vi "FPGA Interleaving.vi"() -> ()   [LabVIEW 2010]
uses:
  <vilib>/LabVIEW Targets/FPGA/cRIO/shared/nicrio_ModuleControls/nicrio_cRIO-9233_DataRatesRing.ctl
  <vilib>/eio/EIOPropertyNode/EIOPropertyNode.xnode
  <vilib>/rvi/eio/nirviEIOPropertyImplementation/nirviEIOPropertyImplementation.xnode
  <vilib>/eio/EIONode/EIONode.xnode
  <vilib>/rvi/eio/nirviEIOImplementation/nirviEIOImplementation.xnode
  <vilib>/rvi/eio/common/nirviEmuClasses.ctl
  <vilib>/rvi/DataTransferAndStorage/Container/XNode/niFpgaContainer.xnode
  <vilib>/rvi/DataTransferAndStorage/Container/Common/niFpgaContainerMethod.ctl
  <vilib>/rvi/DataTransferAndStorage/Container/Common/niFpgaTransferTypeControl.ctl
  <vilib>/rvi/eio/common/nirviEmuTemplatePropertySet_noerrors.vi
  <vilib>/rvi/eio/common/nirviEmuTemplateMethod_noerrors.vi
  <vilib>/rvi/interface/RandomDataEmulation/nirviRandomDataFPGAFIFO.vi
  <vilib>/rvi/interface/RandomDataEmulation/niFpgaRandomDataHandleErrors.vi
panel:
  in  "Samples per Channel":i32
  in  "Data Rate":T1=57 items=["50.000 kS/s (NI 9233)"=2, "33.333 kS/s (NI 9233)"=3, "25.000 kS/s (NI 9233)"=34, "16.667 kS/s (NI 9233)"=35, "12.500 kS/s (NI 9233)"=36, "10.000 kS/s (NI 9233)"=37, "  8.333 kS/s (NI 9233)"=38, "  7.143 kS/s (NI 9233)"=39, "  6.250 kS/s (NI 9233)"=40, "  5.556 kS/s (NI 9233)"=41, "  5.000 kS/s (NI 9233)"=42, "  4.545 kS/s (NI 9233)"=43, "  4.167 kS/s (NI 9233)"=44, "  3.846 kS/s (NI 9233)"=45, "  3.571 kS/s (NI 9233)"=46, "  3.333 kS/s (NI 9233)"=47, "  3.125 kS/s (NI 9233)"=48, "  2.941 kS/s (NI 9233)"=49, "  2.778 kS/s (NI 9233)"=50, "  2.632 kS/s (NI 9233)"=51, "  2.500 kS/s (NI 9233)"=52, "  2.381 kS/s (NI 9233)"=53, "  2.273 kS/s (NI 9233)"=54, "  2.174 kS/s (NI 9233)"=55, "  2.083 kS/s (NI 9233)"=56, "  2.000 kS/s (NI 9233)"=57]
  out "Overflow Occurred":bool
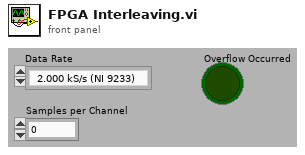
[diagram p1: front panel]
types:
  T1 = typedef "nicrio_cRIO-9233_DataRatesRing.ctl" = u8
  T2 = typedef "nirviEmuClasses.ctl" = enum16{"IO Read", "IO Write", "Method", "Property Read", "Property Write"}
  T3 = typedef "niFpgaContainerMethod.ctl" = enum16{"<none>", "write", "read", "clear", "getNumberOfElementsToWrite", "getNumberOfElementsToRead", "enable", "disable", "flushAndDisable", "getStreamState", "readA", "readB", "dramWrite", "dramWriteWithByteEnables", "dramRequestData", "dramRetrieveData"}
  T4 = typedef "niFpgaTransferTypeControl.ctl" = enum16{"Target-Scoped", "Host to Target - DMA", "Target to Host - DMA", "Peer to Peer Reader", "Peer to Peer Writer", "Bidirectional"}
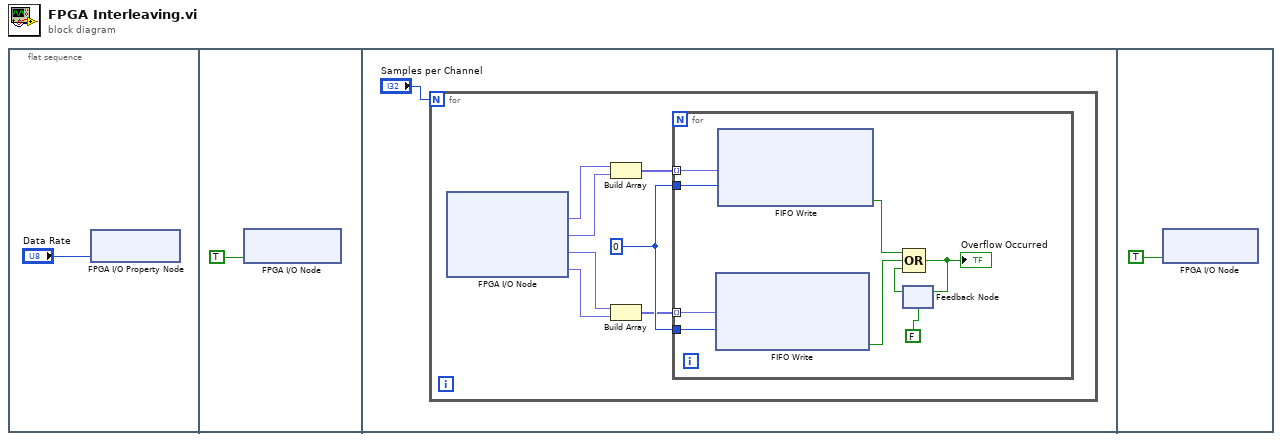
[diagram p0: block diagram]
diagram:
  n1 = flat-sequence {
    frame #0 {
      n2 = xnode "FPGA I/O Property Node"("Data Rate"="Data Rate") -> ()  [unwired: 1 in, 1 out]
    }
    frame #1 {
      n3 = xnode "FPGA I/O Node"("Mod2/Start"=TRUE) -> ()  [unwired: 1 in, 1 out]
    }
    frame #2 {
      n4 = for {
        N: "Samples per Channel" -> [_]
        w27 = 0 ("Timeout")
        n5 = xnode "FPGA I/O Node"() -> ("Accelerometer 0"=w21:fxp<+/-,24,4>, "Accelerometer 1"=w22:fxp<+/-,24,4>, "Thermocouple 0"=w23:fxp<+/-,24,-2>, "Thermocouple 1"=w24:fxp<+/-,24,-2>)  [unwired: 4 in, 4 out]
        n6 = Build Array(w21, w22) -> (w26:fxp<+/-,24,4>[])
        n7 = Build Array(w23, w24) -> (w25:fxp<+/-,24,-2>[])
        n8 = for {
          tunnel: w26 -> [w30] mode=indexing
          tunnel: w27 -> [w36]
          tunnel: w27 -> [w35]
          tunnel: w25 -> [w28] mode=indexing
          n9 = xnode "FIFO Write"("Element"=w28, "Timeout"=w35) -> ("Timed Out?"=w34:bool)  [unwired: 1 in, 1 out]
          n10 = xnode "FIFO Write"("Element"=w30, "Timeout"=w36) -> ("Timed Out?"=w33:bool)  [unwired: 1 in, 1 out]
          n11 = feedback #1(FALSE) -> (w32:bool)
          n12 = Compound Arithmetic op=OR(w33, w34, w32) -> (w31:bool)
          "Overflow Occurred" <- w31
          n13 = feedback-in #1(w31) -> ()
        }
      }
    }
    frame #3 {
      n14 = xnode "FPGA I/O Node"("Mod2/Stop"=TRUE) -> ()  [unwired: 1 in, 1 out]
    }
  }
